vi "Log Text to Sinks.vi"(8 "error in (no error)":errorcluster, 10 "Log Text":string, 11 "Logger in":refnum<class "Logger.lvclass">) -> (0 "error out":errorcluster, 3 "Logger out":refnum<class "Logger.lvclass">)   [LabVIEW 2020, in "LV Log.lvlib" / "Logger.lvclass"]
uses:
  Logger.lvclass
  Logger.lvclass/Logger.ctl
  Sinks/Sink/Sink.lvclass
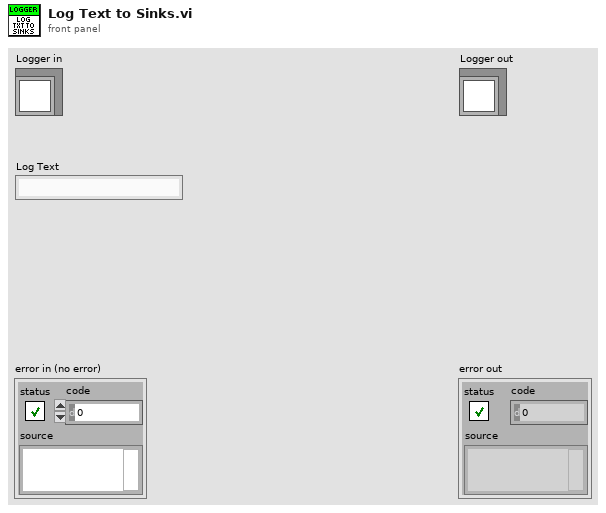
[diagram p1: front panel]
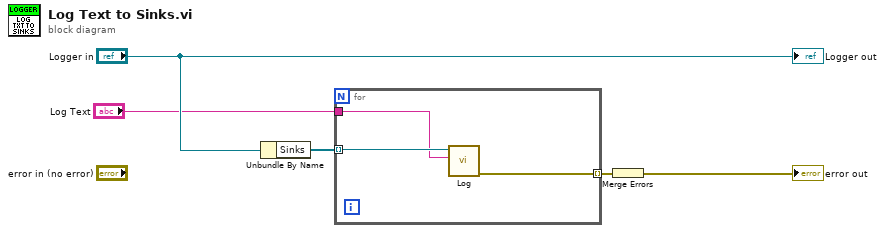
[diagram p0: block diagram]
diagram:
  n1 = Unbundle By Name("Logger in") -> ("Sinks"=w1:refnum<class "Sink.lvclass">[])
  n2 = for {
    tunnel: w1 -> [w8] mode=indexing
    tunnel: "Log Text" -> [w7]
    tunnel: [w6] -> w2 mode=indexing
    n3 = call-dynamic "Log.vi"("Log Text"=w7, "Sink in"=w8) -> ("error out"=w6:errorcluster)  [unwired: 8 in, 1 out]
  }
  n4 = Merge Errors(w2) -> (→"error out":errorcluster)
  "Logger out" <- "Logger in"
